vi "TemperatureLogger.vi"() -> ()   [LabVIEW 2013]
uses:
  <vilib>/Utility/file.llb/Read From Spreadsheet File (DBL).vi
panel:
  out "output cluster":cluster{"all rows":dbl[], "all rows":dbl[]}
  out "XY Chart":cluster{"all rows":dbl[], "all rows":dbl[]}(graph)
  in  "File Path":path
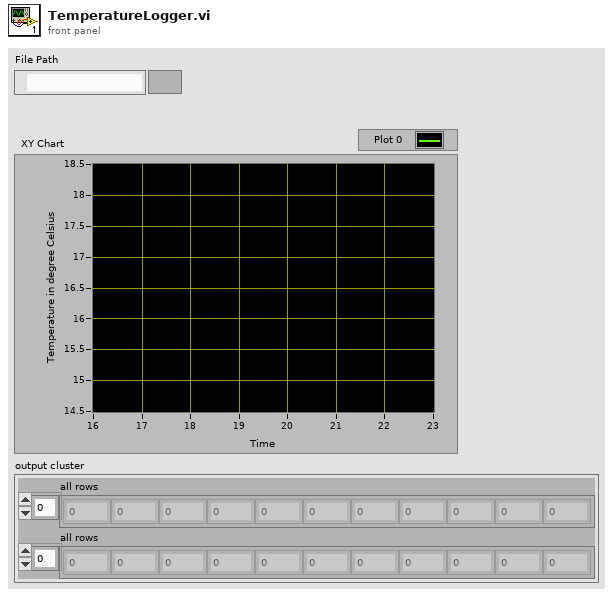
[diagram p1: front panel]
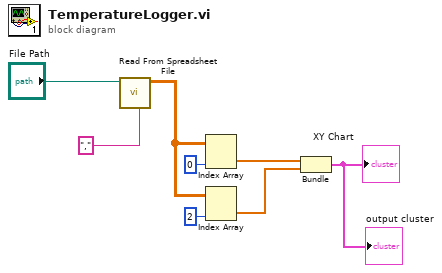
[diagram p0: block diagram]
diagram:
  n1 = call-poly <vilib>:"Read From Spreadsheet File.vi"("delimiter (\\t)"="," ("delimiter (\\t)"), "file path (dialog if empty)"="File Path") -> ("all rows"=w1:dbl[][])  [unwired: 5 in, 4 out]
  n2 = Index Array(array=w1, index (col)=0 ("disabled index (col)")) -> (element=w4:dbl[])  [unwired: 1 in]
  n3 = Index Array(array=w1, index (col)=2 ("disabled index (col)")) -> (element=w3:dbl[])  [unwired: 1 in]
  n4 = Bundle("all rows"=w4, "all rows"=w3) -> (→"XY Chart" →"output cluster":cluster{"all rows":dbl[], "all rows":dbl[]})  [unwired: 1 in]
